vi "RGA_scan_new_version.vi"() -> ()   [LabVIEW 2018]
panel:
  out "Average Press [Torr]":dbl
  in  "Run Scan":bool
  out "1 Torr Baratron [Torr]":dbl format="%#_13g"
  out "String":string
  in  "Number of Scans":string
  in  "Detector Index":string
  in  "Source Index":string
  in  "E Gain Index":string
  in  "Accuracy":string
  in  "Points Per Peak":string
  in  "End Mass":string
  in  "Start Mass":string
  in  "Measurement Name":string
  out "standard error":string
  out "standard output":string
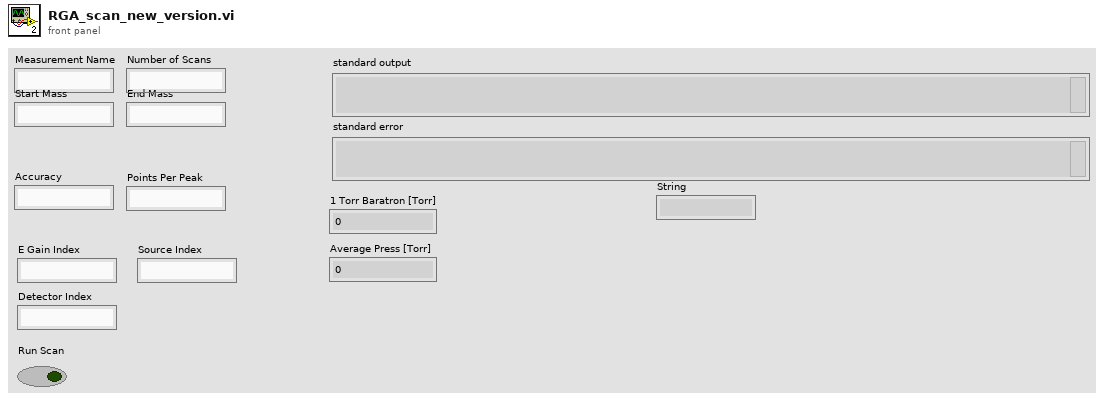
[diagram p1: front panel]
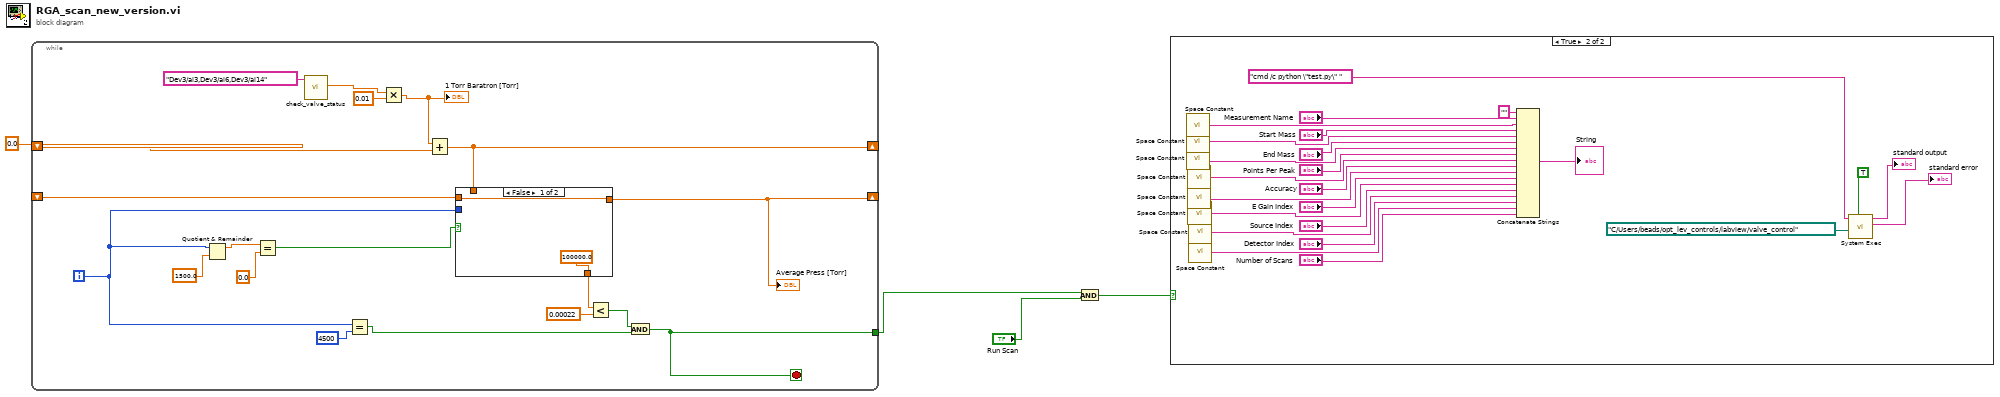
[diagram p0: block diagram]
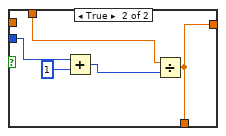
[diagram p2: hidden frame]
diagram:
  n1 = while {
    shift-right: [w18] -> _
    shift-left: 0.0 -> [w19]
    shift-right: [w12] -> _
    shift-left: _ -> [w17]
    tunnel: [w5] -> w1
    i -> [w11]
    stop <- w5 stop-if-true
    n2 = Quotient & Remainder(x=w11, y=1500.0) -> (x-y*floor(x/y)=w15:dbl)  [unwired: 1 out]
    n3 = Equal?(x=w15, y=0.0) -> (x = y?=w13:bool)
    n4 = call "check_valve_status.vi"("Channel 1"=tag "Dev3/ai3,Dev3/ai6,Dev3/ai14") -> ("Ch. 2 value"=w21:dbl)  [unwired: 8 in, 2 out]
    n5 = Equal?(x=w11, y=4500) -> (x = y?=w9:bool)
    n6 = Multiply(x=w21, y=0.01) -> (x*y=w20:dbl)
    "1 Torr Baratron [Torr]" <- w20
    n7 = Add(x=w20, y=w19) -> (x+y=w18:dbl)
    n8 = case shown="False" w13 {
      tunnel: w11 -> [_ w30]
      tunnel: w18 -> [_ w28]
      tunnel: [w25 w26] -> w12
      tunnel: w17 -> [w25 _]
      tunnel: [100000.0 w26] -> w8
      frame False {
      }
      frame True {
        n9 = Add(x=w30, y=1) -> (x+y=w27:i32)
        n10 = Divide(x=w28, y=w27) -> (x/y=w26:dbl)
      }
    }
    "Average Press [Torr]" <- w12
    n11 = Less?(x=w8, y=0.00022) -> (x < y?=w6:bool)
    n12 = And(x=w6, y=w9) -> (x .and. y?=w5:bool)
  }
  n13 = And(x=w1, y="Run Scan") -> (x .and. y?=w4:bool)
  n14 = case shown="True" w4 {
    frame False {
    }
    frame True {
      n15 = call <vilib>:"Space Constant.vi"() -> ("String"=w49:string)
      n16 = call <vilib>:"Space Constant.vi"() -> ("String"=w47:string)
      n17 = call <vilib>:"Space Constant.vi"() -> ("String"=w45:string)
      n18 = call <vilib>:"Space Constant.vi"() -> ("String"=w43:string)
      n19 = call <vilib>:"Space Constant.vi"() -> ("String"=w41:string)
      n20 = call <vilib>:"Space Constant.vi"() -> ("String"=w39:string)
      n21 = call <vilib>:"Space Constant.vi"() -> ("String"=w37:string)
      n22 = call <vilib>:"Space Constant.vi"() -> ("String"=w35:string)
      n23 = Concatenate Strings("" ("string"), "Measurement Name", w49, "Start Mass", w47, "End Mass", w45, "Points Per Peak", w43, "Accuracy", w41, "E Gain Index", w39, "Source Index", w37, "Detector Index", w35, "Number of Scans") -> (→"String":string)
      n24 = call <vilib>:"System Exec.vi"("wait until completion? (T)"=TRUE, "working directory"=path "C:/Users/beads/opt_lev_controls/labview/valve_control", "command line"="cmd /c python \"test.py\" ") -> ("standard error"=→"standard error":string, "standard output"=→"standard output":string)  [unwired: 5 in, 2 out]
    }
  }
